vi "Processing.GUI.vi"(8 "error in":errorcluster) -> ()   [LabVIEW 2019, in "Tools.lvlib"]
uses:
  Tools.lvlib
panel:
  out "error out":errorcluster
  in  "stop":bool
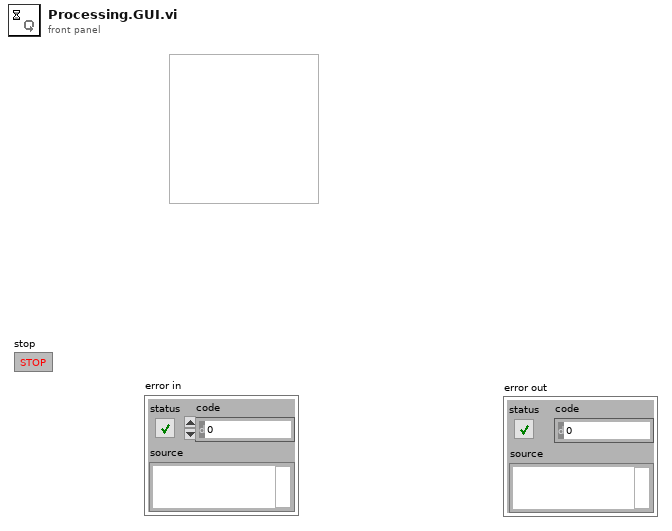
[diagram p1: front panel]
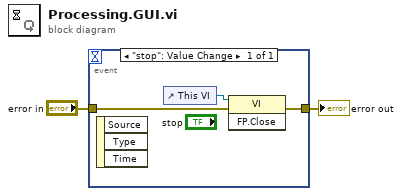
[diagram p0: block diagram]
diagram:
  n1 = event shown="[0] \"stop\": Value Change" {
    selector: _ -> [_]
    dyn-events: _ -> [_]
    timeout: _ -> [_]
    tunnel: "error in" -> [w4]
    tunnel: [w3] -> w1
    event "stop": Value Change {
      n2 = event-data() -> ()  [unwired: 1 in, 3 out]
      n3 = control-ref of="This VI"() -> (w5:refnum<vi>)
      n4 = invoke class="VI" method="FP.Close"(reference=w5, error in=w4) -> (error out=w3:errorcluster)  [unwired: 1 in, 2 out]
    }
  }
  "error out" <- w1
